vi "Destroy Self.vi"(7 "Sender":refnum<class "Sender.lvclass">, 11 "Base Actor in":refnum<class "Base Actor.lvclass">) -> (0 "Error out":errorcluster, 3 "Base Actor out":refnum<class "Base Actor.lvclass">)   [LabVIEW 2025, in "jettl.lvlib" / "Actor.lvlib" / "Base Actor.lvclass"]
uses:
  Base Actor.lvclass
  Sender/Sender/Sender.lvclass
  Base Actor.lvclass/Base Actor.ctl
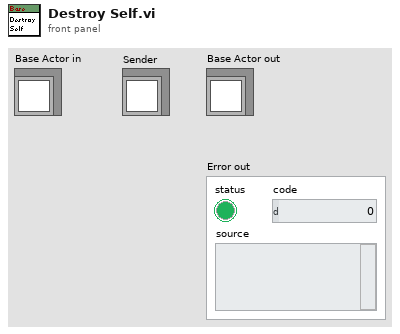
[diagram p1: front panel]
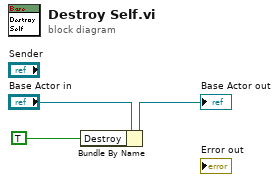
[diagram p0: block diagram]
diagram:
  n1 = Bundle By Name(cluster="Base Actor in", "Destroy"=TRUE ("Is Marked For Destroy")) -> (→"Base Actor out":refnum<class "Base Actor.lvclass">)
